vi "Woodhouse.vi"(11 "Files in":T1[](array[typedef])) -> (3 "Files out":T1[](array[typedef]))   [LabVIEW 2022 SP3]
uses:
  Curtin1_Label.ctl
panel:
  out "Graph":dbl[](graph)
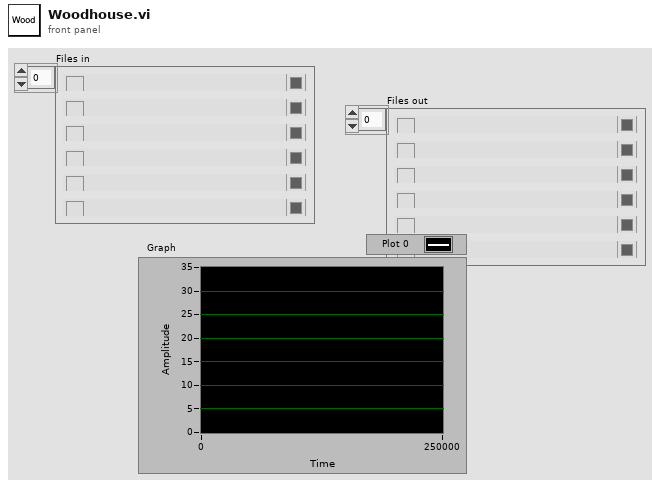
[diagram p1: front panel]
types:
  T1 = typedef "Curtin1_Label.ctl" = cluster{"Show?":bool, "Name":string, "Color":u32, "Path":path, "Show Notes":bool}
  T2 = enum16{"big-endian, network order", "native, host order", "little-endian"}
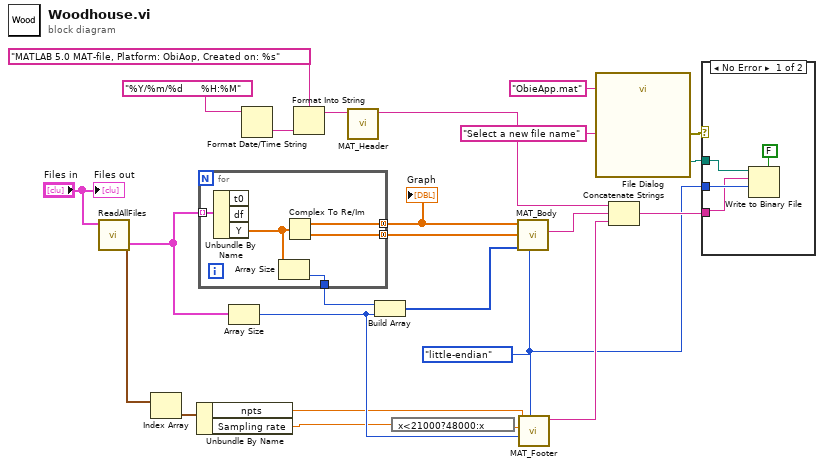
[diagram p0: block diagram]
diagram:
  w8 = T2."little-endian" ("byte order (0:big-endian, network order)")
  n1 = call "ReadAllFiles.vi"("Files"="Files in") -> ("info"=w6:cluster{"Sampling rate":dbl, "npts":dbl}[], "data"=w21:cluster{"t0":dbl, "df":dbl, "Y":cdb[]}[])  [unwired: 5 in, 4 out]
  n2 = Index Array(array=w6) -> (element=w5:cluster{"Sampling rate":dbl, "npts":dbl})  [unwired: 1 in]
  n3 = Unbundle By Name(w5) -> ("npts"=w2:dbl, "Sampling rate"=w4:dbl)
  n4 = for {
    tunnel: w21 -> [w30] mode=indexing
    tunnel: [w29] -> w3
    tunnel: [w28] -> w9 mode=concatenating
    tunnel: [w27] -> w18 mode=concatenating
    n5 = Unbundle By Name(w30) -> ("Y"=w26:cdb[])  [unwired: 2 out]
    n6 = Array Size(array=w26) -> (size(s)=w29:i32)
    n7 = Complex To Re/Im(x + iy=w26) -> (x=w27:dbl[], y=w28:dbl[])
  }
  "Graph" <- w18
  n8 = Array Size(array=w21) -> (size(s)=w14:i32)
  n9 = Format Date/Time String(time format string (%c)="%Y/%m/%d      %H:%M") -> (date/time string=w23:string)  [unwired: 2 in]
  n10 = Format Into String(format string="MATLAB 5.0 MAT-file, Platform: ObiAop, Created on: %s" ("Title"), w23) -> (resulting string=w20:string)  [unwired: 2 in, 1 out]
  n11 = call "MAT_Header.vi"("Title String"=w20) -> ("String out"=w16:string)  [unwired: 10 in]
  n12 = Build Array(w3, w14) -> (w7:i32[])
  n13 = expression code="x<21000?48000:x"(w4) -> (w1:dbl)
  n14 = call "MAT_Body.vi"("byte order"=w8, "Dimensions"=w7, "Imag"=w9, "Real"=w18) -> ("String Out"=w15:string)  [unwired: 6 in, 1 out]
  n15 = call "MAT_Footer.vi"("byte order"=w8, "# plots"=w14, "frequency"=w1, "npts"=w2) -> ("String"=w17:string)  [unwired: 7 in]
  n16 = call "File Dialog"("prompt"="Select a new file name", "default name"="ObieApp.mat") -> ("selected path"=w11:path, "error out"=w10:errorcluster)  [unwired: 10 in, 2 out]
  n17 = Concatenate Strings(w16, w15, w17) -> (w19:string)
  n18 = case shown="No Error" w10 {
    tunnel: w19 -> [w31 _]
    tunnel: w8 -> [w33 _]
    tunnel: w11 -> [w32 _]
    frame No Error {
      n19 = Write to Binary File(file (use dialog)=w32, data=w31, 5:FALSE ("prepend array or string size? (T)"), 9:w33) -> ()  [unwired: 2 in, 3 out]
    }
    frame Error {
    }
  }
  "Files out" <- "Files in"
